vi "ScopeSubVI.vi"(9 "error in":errorcluster, 10 "trigger level":dbl=-0.05, 11 "instrument handle":refnum<k15>) -> (1 "wfm":waveform(dbl), 2 "error out":errorcluster, 3 "instrument handle out":refnum<k15>)   [LabVIEW 2012]
uses:
  <instrlib>/niScope/Controls/niScope trigger source.ctl
  <instrlib>/niScope/Controls/niScope trigger slope.ctl
  <instrlib>/niScope/Configure/Trigger/niScope Configure Trigger Edge.vi
  <instrlib>/niScope/Acquire/niScope Read WDT.vi
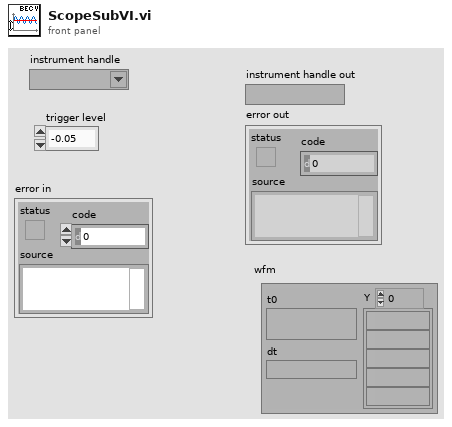
[diagram p1: front panel]
types:
  T1 = typedef "niScope trigger slope.ctl" = i32
  T2 = typedef "niScope trigger source.ctl" = string
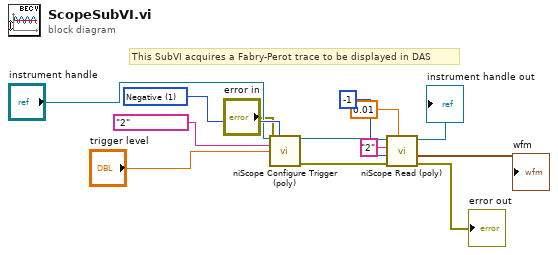
[diagram p0: block diagram]
diagram:
  w10 = T1 1 items=["Positive", "Negative"] ("trigger slope")
  # "This SubVI acquires a Fabry-Perot trace to be displayed in DAS"
  n1 = call-poly <instrlib>:"niScope Configure Trigger (poly).vi"("instrument handle"="instrument handle", "trigger slope"=w10, "trigger source"=T2 "2", "trigger level"="trigger level", "error in"="error in") -> ("instrument handle out"=w12:refnum<k15>, "error out"=w11:errorcluster)  [unwired: 9 in]
  n2 = call-poly <instrlib>:"niScope Read (poly).vi"("timeout"=0.01, "error in"=w11, "numSamples"=-1, "channels"="2", "instrument handle"=w12) -> ("error out"=→"error out":errorcluster, "wfm"=→"wfm":waveform(dbl), "instrument handle out"=→"instrument handle out":refnum<k15>)  [unwired: 3 in, 1 out]
